vi "Read Channel State.vi"(8 "error in (no error)":errorcluster, 11 "Channel in":refnum<class "Channel.lvclass">) -> (0 "error out":errorcluster, 2 "State":T1, 3 "Channel out":refnum<class "Channel.lvclass">)   [LabVIEW 2020, in "G-Audio.lvlib" / "Channel.lvclass"]
uses:
  Channel.lvclass
  5f550c92-b999-4666-ba10-b652889d4234.vi
  Channel State.ctl
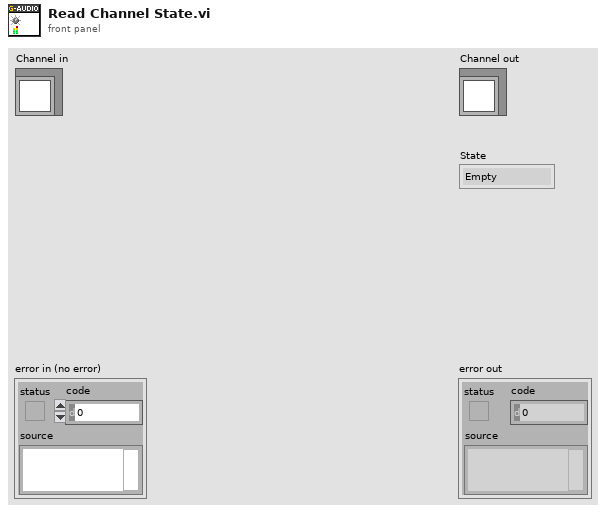
[diagram p1: front panel]
types:
  T1 = typedef "G-Audio.lvlib/Channel.lvclass/Channel State.ctl" = enum16{"Empty", "Loading", "Stopped", "Paused", "Playing", "Retrigger"}
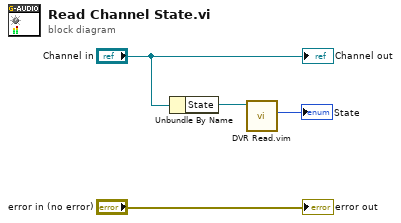
[diagram p0: block diagram]
diagram:
  n1 = Unbundle By Name("Channel in") -> ("State"=w4:refnum<data-value>)
  n2 = call "DVR Read.vim"("DVR In"=w4) -> ("Data"=→"State":T1)  [unwired: 9 in, 1 out]
  "error out" <- "error in (no error)"
  "Channel out" <- "Channel in"
